vi "myRIO_BRig_Host_parse_dataBlock__v3.vi"(10 "input_dataCurrent":u16[](array[numeric]), 11 "input_dataBlock":u16[][](array[numeric])) -> (0 "BlockR_T2R_avg":dbl caption="Trials2Reward", 1 "BlockR_BTPR_avg":dbl caption="BadTrialsPostReward", 2 "BlockL_BTPR_avg":dbl caption="BadTrialsPostReward" format="%#_3g", 3 "BlockL_T2R_avg":dbl caption="Trials2Reward" format="%#_3g", 4 "BlockR_BTPR_cur":u16 caption="BadTrialsPostReward", 5 "BlockL_BTPR_cur":u16 caption="BadTrialsPostReward", 6 "BlockR_T2R_cur":u16 caption="Trials2Reward", 7 "BlockL_T2R_cur":u16 caption="Trials2Reward")   [LabVIEW 2014]
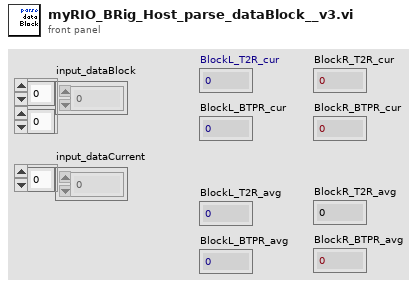
[diagram p1: front panel]
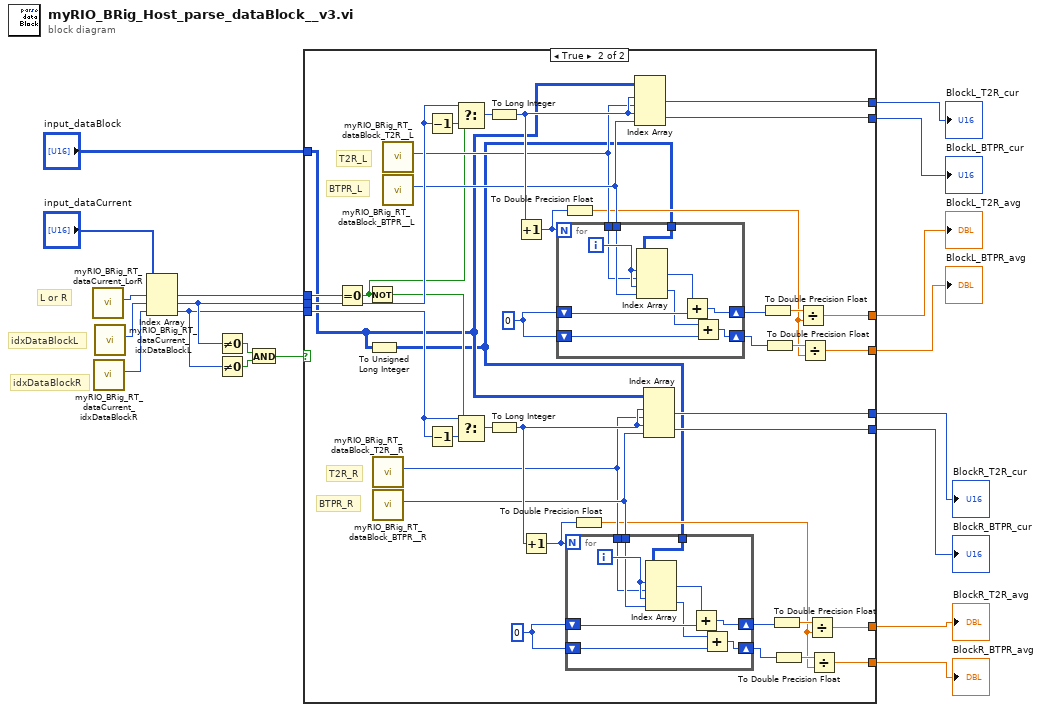
[diagram p0: block diagram]
diagram:
  # "L or R"
  # "idxDataBlockR"
  # "idxDataBlockL"
  n1 = call "myRIO_BRig_RT_dataCurrent_LorR.vi"() -> ("output_LorR"=w17:i32)  [unwired: 11 in]
  n2 = call "myRIO_BRig_RT_dataCurrent_idxDataBlockR.vi"() -> ("output_idxDataBlock__R"=w1:i32)  [unwired: 11 in]
  n3 = call "myRIO_BRig_RT_dataCurrent_idxDataBlockL.vi"() -> ("output_idxDataBlock__L"=w18:i32)  [unwired: 11 in]
  n4 = Index Array(array="input_dataCurrent", index #1=w17, index #2=w18, index #3=w1) -> (element #1=w12:u16, element #2=w11:u16, element #3=w10:u16)
  n5 = Not Equal To 0?(x=w11) -> (x != 0?=w15:bool)
  n6 = Not Equal To 0?(x=w10) -> (x != 0?=w16:bool)
  n7 = And(x=w15, y=w16) -> (x .and. y?=w14:bool)
  n8 = case shown="True" w14 {
    tunnel: "input_dataBlock" -> [_ w21]
    tunnel: w12 -> [_ w29]
    tunnel: w11 -> [_ w57]
    tunnel: w10 -> [_ w26]
    tunnel: [_ w55] -> w7
    tunnel: [_ w54] -> w6
    tunnel: [_ w47] -> w9
    tunnel: [_ w42] -> w8
    tunnel: [_ w25] -> w3
    tunnel: [_ w24] -> w2
    tunnel: [_ w23] -> w4
    tunnel: [_ w22] -> w5
    frame False {
    }
    frame True {
      w36 = u32 0
      w50 = u32 0
      # "BTPR_R"
      # "T2R_R"
      # "BTPR_L"
      # "T2R_L"
      n9 = Equal To 0?(x=w29) -> (x = 0?=w28:bool)
      n10 = Not(x=w28) -> (.not. x?=w27:bool)
      n11 = To Unsigned Long Integer(number=w21) -> (unsigned 32bit integer=w20:u32[][])
      n12 = call "myRIO_BRig_RT_dataBlock_T2R__R.vi"() -> ("output_T2R__R"=w37:i32)  [unwired: 11 in]
      n13 = call "myRIO_BRig_RT_dataBlock_BTPR__R.vi"() -> ("output_BTPR__R"=w38:i32)  [unwired: 11 in]
      n14 = call "myRIO_BRig_RT_dataBlock_T2R__L.vi"() -> ("output_T2R__L"=w51:i32)  [unwired: 11 in]
      n15 = call "myRIO_BRig_RT_dataBlock_BTPR__L.vi"() -> ("output_BTPR__L"=w52:i32)  [unwired: 11 in]
      n16 = Decrement(x=w57) -> (x-1=w58:u16)
      n17 = Decrement(x=w26) -> (x-1=w41:u16)
      n18 = Select(t=w57, s=w28, f=w58) -> (s? t:f=w56:u16)
      n19 = Select(t=w26, s=w27, f=w41) -> (s? t:f=w40:u16)
      n20 = To Long Integer(number=w56) -> (32bit integer=w53:i32)
      n21 = To Long Integer(number=w40) -> (32bit integer=w39:i32)
      n22 = Increment(x=w53) -> (x+1=w45:i32)
      n23 = Increment(x=w39) -> (x+1=w32:i32)
      n24 = for {
        N: w45 -> [_]
        tunnel: w52 -> [w77]
        tunnel: w51 -> [w76]
        shift-right: [w72] -> w48
        shift-left: w50 -> [w73]
        shift-right: [w75] -> w43
        shift-left: w50 -> [w74]
        tunnel: w20 -> [w71]
        i -> [w78]
        n25 = Index Array(array=w71, index (row) #1=w78, index (col) #1=w76, index (row) #2=w78, index (col) #2=w77) -> (element #1=w70:u32, element #2=w69:u32)
        n26 = Add(x=w70, y=w73) -> (x+y=w72:u32)
        n27 = Add(x=w69, y=w74) -> (x+y=w75:u32)
      }
      n28 = To Double Precision Float(number=w45) -> (double precision float=w44:dbl)
      n29 = for {
        N: w32 -> [_]
        tunnel: w38 -> [w67]
        tunnel: w37 -> [w66]
        shift-right: [w62] -> w34
        shift-left: w36 -> [w63]
        shift-right: [w65] -> w30
        shift-left: w36 -> [w64]
        tunnel: w20 -> [w61]
        i -> [w68]
        n30 = Index Array(array=w61, index (row) #1=w68, index (col) #1=w66, index (row) #2=w68, index (col) #2=w67) -> (element #1=w59:u32, element #2=w60:u32)
        n31 = Add(x=w59, y=w63) -> (x+y=w62:u32)
        n32 = Add(x=w60, y=w64) -> (x+y=w65:u32)
      }
      n33 = To Double Precision Float(number=w32) -> (double precision float=w31:dbl)
      n34 = Index Array(array=w21, index (row) #1=w53, index (col) #1=w51, index (row) #2=w53, index (col) #2=w52) -> (element #1=w55:u16, element #2=w54:u16)
      n35 = Index Array(array=w21, index (row) #1=w39, index (col) #1=w37, index (row) #2=w39, index (col) #2=w38) -> (element #1=w25:u16, element #2=w24:u16)
      n36 = To Double Precision Float(number=w48) -> (double precision float=w49:dbl)
      n37 = To Double Precision Float(number=w43) -> (double precision float=w46:dbl)
      n38 = To Double Precision Float(number=w34) -> (double precision float=w35:dbl)
      n39 = To Double Precision Float(number=w30) -> (double precision float=w33:dbl)
      n40 = Divide(x=w49, y=w44) -> (x/y=w47:dbl)
      n41 = Divide(x=w46, y=w44) -> (x/y=w42:dbl)
      n42 = Divide(x=w35, y=w31) -> (x/y=w22:dbl)
      n43 = Divide(x=w33, y=w31) -> (x/y=w23:dbl)
    }
  }
  "BlockR_T2R_avg" <- w5
  "BlockR_BTPR_avg" <- w4
  "BlockR_T2R_cur" <- w3
  "BlockR_BTPR_cur" <- w2
  "BlockL_T2R_avg" <- w9
  "BlockL_BTPR_avg" <- w8
  "BlockL_T2R_cur" <- w7
  "BlockL_BTPR_cur" <- w6
